vi "Unibot - Nonlinear Model 2.vi"(4 "Amplifier Gain":dbl(slide)=1.0 scale=-0.1..0.1, 6 "Torque (Tau)":dbl=1.0, 9 "Moment of Inetia of the frame wrt to center of mass (Ifg)":dbl=20.0, 10 "Distance from center of wheel to center of mass (Rf)":dbl=0.463, 11 "Mass of Frame (mf)":dbl=25.0) -> (0 "xPos1":dbl=-0.3578561321200968, 1 "alpha1":dbl=0.11676928692181643, 2 "states":dbl[](array[numeric]))   [LabVIEW 2012]
uses:
  <vilib>/Simulation/Implementation/Shared/SIMSCR Execution Mode.ctl
  <vilib>/Simulation/Scripting/Companion Diagram/SimConfigNode/SimParams.ctl
  <vilib>/Simulation/Scripting/Companion Diagram/SimConfigNode/_simSolvers.ctl
  <vilib>/Simulation/Param Hierarchy/Typedefs/SIMPH Param Control Actions.ctl
  <vilib>/Simulation/Implementation/Shared/SIM limit type.ctl
  <vilib>/Simulation/Implementation/Shared/NILVSim_ParamChanged.vi
  <vilib>/Simulation/ContinuousLinear/Implementation/NILVSim Integrator new.llb/SIM Integrator distributor (scalar).vi
  <vilib>/Simulation/ContinuousLinear/Implementation/NILVSim Integrator new.llb/SIM Integrator collector (scalar).vi
  <vilib>/Simulation/Implementation/Shared/NILVSim_Manager.vi
  <vilib>/Simulation/Implementation/Shared/NILVSim_FinalizeModel.vi
  <vilib>/Simulation/Implementation/Shared/SIM Unbundle Sim Info.vi
  <vilib>/Utility/error.llb/Clear Errors.vi
  <vilib>/Simulation/Implementation/Shared/NILVSim_GetModelError.vi
  <vilib>/Simulation/Implementation/Shared/SIM SimErrorHandler.vi
  <vilib>/Simulation/Implementation/Shared/SIM Bundle Sim Info.vi
  <vilib>/Simulation/Implementation/Shared/SIMSH Read Queue.vi
  <vilib>/Simulation/Implementation/Shared/NILVSim_Initialize.vi
  <vilib>/Simulation/Utility/Implementation/NILVSim Get Time and IsAcceptedStep.vi
  <vilib>/Simulation/Scripting/Companion Diagram/SimConfigNode/SimDog.xnode
  <vilib>/Simulation/Implementation/XNodeFramework/SimXNode/SimX.xnode
  <vilib>/Simulation/ContinuousLinear/Implementation/NILVSim Integrator new.llb/SIM Integrator (scalar).vi
  <vilib>/ptbypt/NI_PtbyPt.lvlib
  <vilib>/Simulation/Implementation/Shared/NI_SIM_Implementation.lvlib
panel:
  in  "initial x position":dbl
  in  "initial x velocity":dbl
  in  "initial velocity alpha":dbl
  in  "initial alpha":dbl=3.14159
  # "Legend: \nC.G.  - Center of Gravity\nl       - Length (m)\nJ      - Moment of Inertia (kg(m^2)\nM     - Mass (kg)"
  # "Derived Parameters"
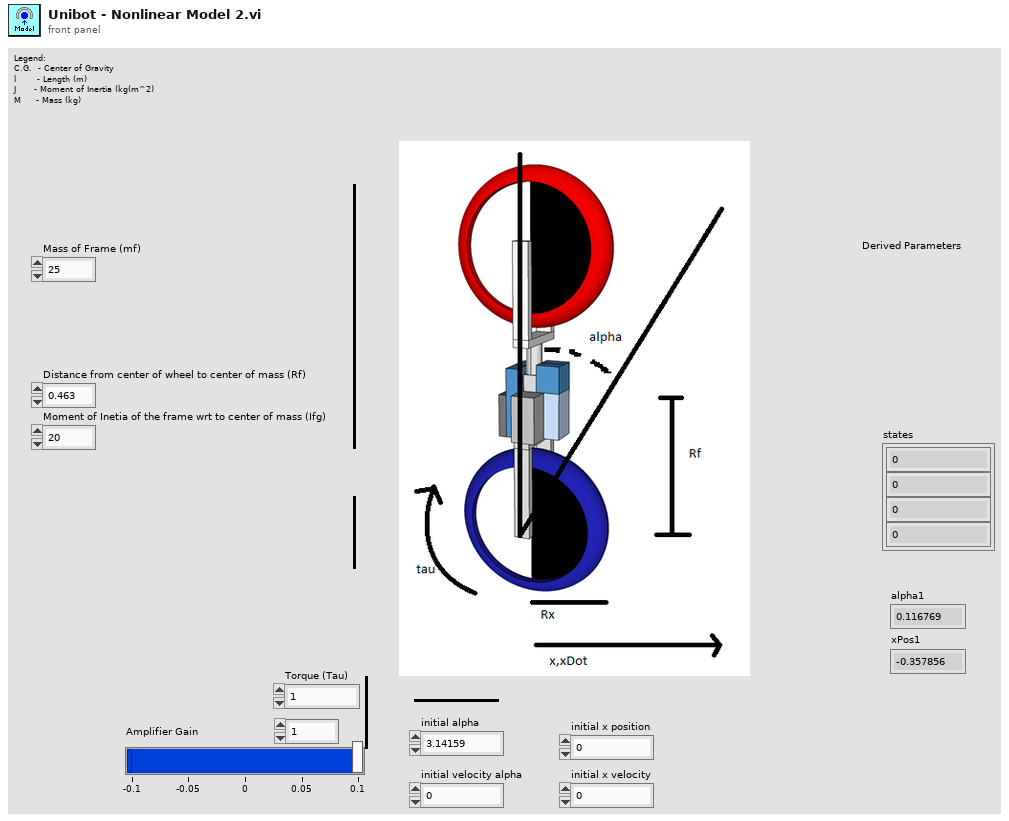
[diagram p1: front panel]
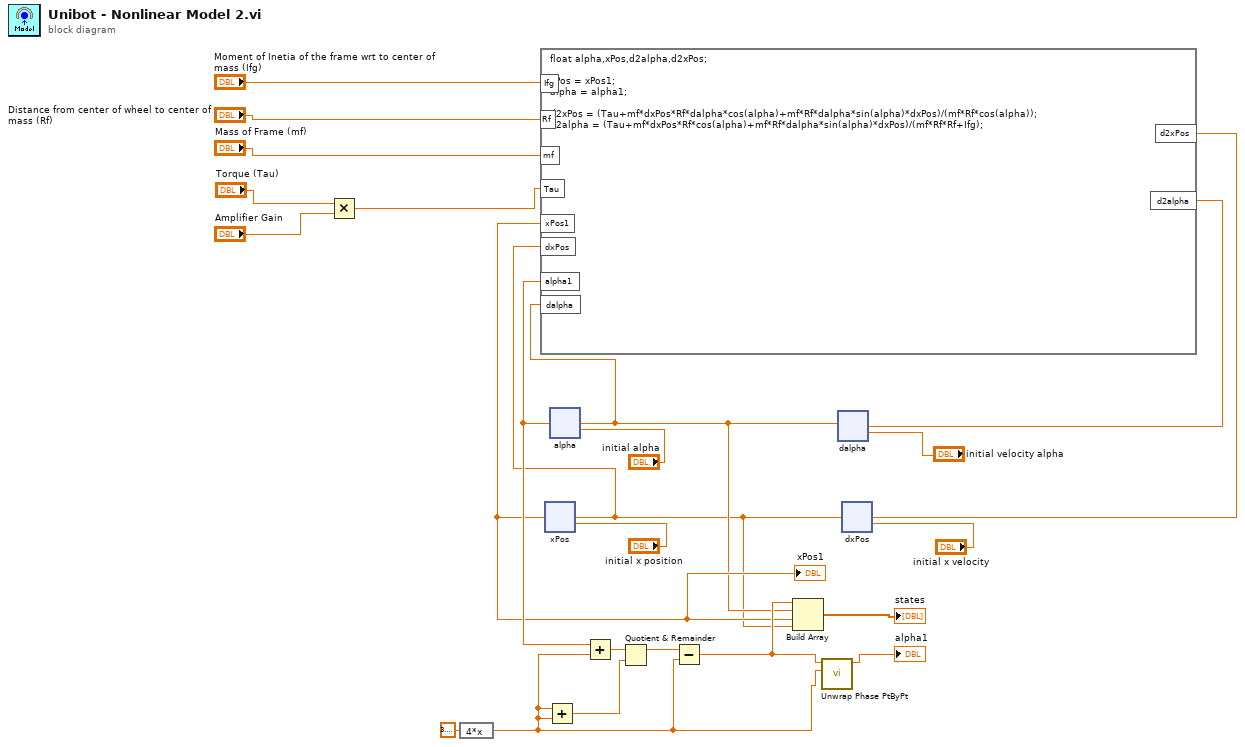
[diagram p0: block diagram]
diagram:
  n1 = Multiply ("Multiply 8")(x="Torque (Tau)", y="Amplifier Gain") -> (x*y=w19:dbl)
  n2 = expression code="4*x"(3.141592653589793 ("Constant")) -> (w10:dbl)
  n3 = Add ("Add 6")(x=w10, y=w10) -> (x+y=w12:dbl)
  n4 = formula code="float alpha,xPos,d2alpha,d2xPos;\n\nxPos = xPos1;\nalpha = alpha1;\n\nd2xPos = (Tau+mf*dxPos*Rf*dalpha*cos(alpha)+mf*Rf*dalpha*sin(alpha)*dxPos)/(mf*Rf*cos(alpha));\nd2alpha = (Tau+mf*dxPos*Rf*cos(alpha)+mf*Rf*dalpha*sin(alpha)*dxPos)/(mf*Rf*Rf+Ifg);" ("Formula Node 2")("Ifg"="Moment of Inetia of the frame wrt to center of mass (Ifg)", "Rf"="Distance from center of wheel to center of mass (Rf)", "mf"="Mass of Frame (mf)", "Tau"=w19, "alpha1"=w5, "dalpha"=w3, "dxPos"=w2, "xPos1"=w4) -> ("d2alpha"=w18:dbl, "d2xPos"=w1:dbl)
  n5 = xnode "dalpha"("input"=w18, "initial condition"="initial velocity alpha") -> ("output"=w3:dbl)  [unwired: 8 in, 2 out]
  n6 = xnode "alpha"("input"=w3, "initial condition"="initial alpha") -> ("output"=w5:dbl)  [unwired: 8 in, 2 out]
  n7 = Add ("Add 5")(x=w5, y=w10) -> (x+y=w14:dbl)
  n8 = Quotient & Remainder ("Quotient & Remainder 2")(x=w14, y=w12) -> (x-y*floor(x/y)=w15:dbl)  [unwired: 1 out]
  n9 = Subtract ("Subtract 2")(x=w15, y=w10) -> (x-y=w8:dbl)
  n10 = call <vilib>:"Unwrap Phase PtByPt.vi"("wrap base"=w10, "phase"=w8) -> ("unwrapped phase"=→"alpha1":dbl)  [unwired: 9 in]
  n11 = xnode "dxPos"("input"=w1, "initial condition"="initial x velocity") -> ("output"=w2:dbl)  [unwired: 8 in, 2 out]
  n12 = xnode "xPos"("input"=w2, "initial condition"="initial x position") -> ("output"=w4:dbl)  [unwired: 8 in, 2 out]
  "xPos1" <- w4
  n13 = Build Array(w8, w3, w4, w2) -> (→"states":dbl[])
